vi "disp_dual.vi"(6 "I_B":dbl(slide) scale=0.1..100.0, 7 "I_A":dbl(slide) scale=0.1..100.0, 9 "img_CHB":sgl[][](graph)=array256x256[65536 elements], 10 "img_CHA":sgl[][](graph)=array256x256[65536 elements], 11 "Image Dst":T1) -> (3 "Image":T1(plugin-control))   [LabVIEW 2015]
uses:
  <vilib>/vision/Image Controls.llb/IMAQ Image.ctl
  <vilib>/vision/NI_Vision_Development_Module.lvlib
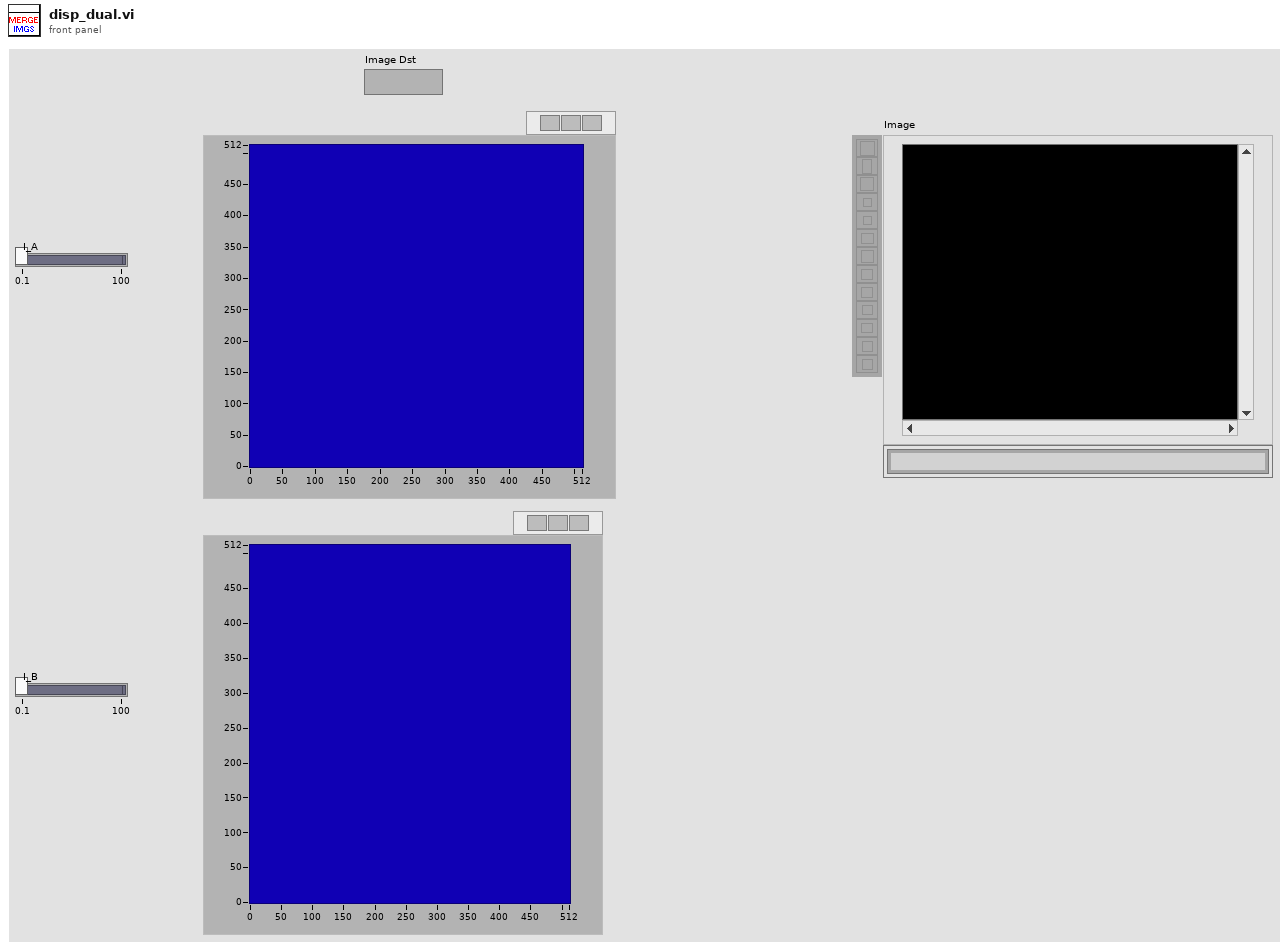
[diagram p1: front panel]
types:
  T1 = typedef "IMAQ Image.ctl" = refnum<image>
  T2 = typedef "Image Type" = u32
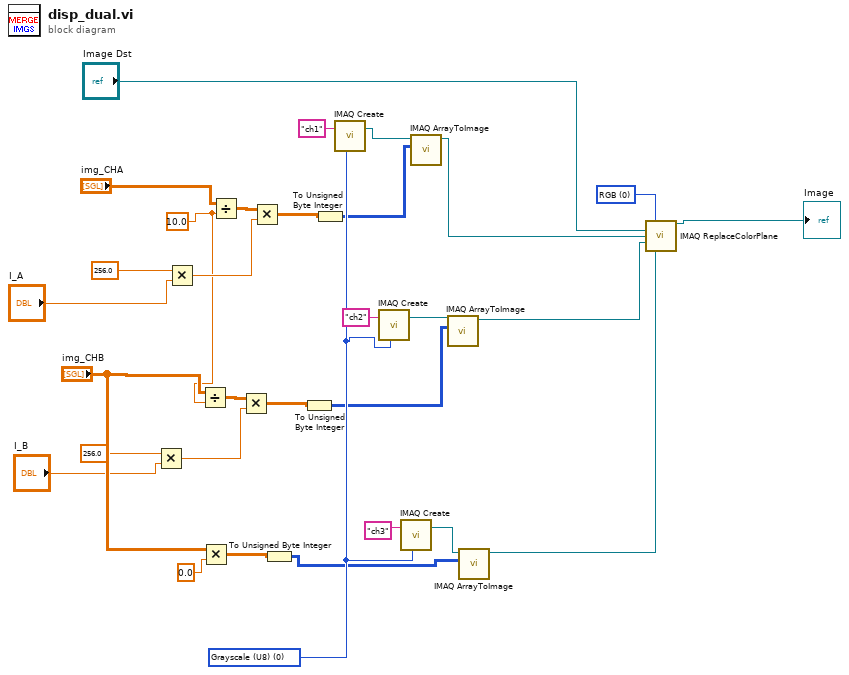
[diagram p0: block diagram]
diagram:
  w1 = 10.0 ("y")
  w21 = T2 0 items=["Grayscale (U8)", "Grayscale (I16)", "Grayscale (SGL)", "Complex (CSG)", "RGB (U32)", "HSL (U32)", "RGB (U64)", "Grayscale (U16)"] ("Image Type")
  w31 = u16 0 items=["RGB", "HSL", "HSV", "HSI"] ("Color Mode")
  n1 = Multiply(x=256.0 ("y"), y="I_B") -> (x*y=w2:dbl)
  n2 = Multiply(x=256.0 ("y"), y="I_A") -> (x*y=w6:dbl)
  n3 = Divide(x="img_CHB", y=w1) -> (x/y=w20:dbl[][])
  n4 = Multiply(x="img_CHB", y=0.0) -> (x*y=w17:dbl[][])
  n5 = Divide(x="img_CHA", y=w1) -> (x/y=w23:dbl[][])
  n6 = Multiply(x=w20, y=w2) -> (x*y=w19:dbl[][])
  n7 = Multiply(x=w23, y=w6) -> (x*y=w22:dbl[][])
  n8 = To Unsigned Byte Integer(number=w17) -> (unsigned 8bit integer=w11:u8[][])
  n9 = To Unsigned Byte Integer(number=w19) -> (unsigned 8bit integer=w9:u8[][])
  n10 = To Unsigned Byte Integer(number=w22) -> (unsigned 8bit integer=w10:u8[][])
  n11 = call "IMAQ Create"("Image Name"="ch1", "Image Type"=w21) -> ("New Image"=w29:T1)  [unwired: 3 in, 1 out]
  n12 = call "IMAQ Create"("Image Name"="ch2", "Image Type"=w21) -> ("New Image"=w28:T1)  [unwired: 3 in, 1 out]
  n13 = call "IMAQ Create"("Image Name"="ch3", "Image Type"=w21) -> ("New Image"=w18:T1)  [unwired: 3 in, 1 out]
  n14 = call "IMAQ ArrayToImage"("Image Pixels (U8)"=w10, "Image"=w29) -> ("Image Out"=w15:T1)  [unwired: 8 in, 1 out]
  n15 = call "IMAQ ArrayToImage"("Image Pixels (U8)"=w9, "Image"=w28) -> ("Image Out"=w14:T1)  [unwired: 8 in, 1 out]
  n16 = call "IMAQ ArrayToImage"("Image Pixels (U8)"=w11, "Image"=w18) -> ("Image Out"=w13:T1)  [unwired: 8 in, 1 out]
  n17 = call "IMAQ ReplaceColorPlane"("Color Mode"=w31, "Image Dst"="Image Dst", "Red or Hue Plane"=w15, "Green or Sat Plane"=w14, "Blue or Luma or Val or Inten Plane"=w13) -> ("Image Dst Out"=→"Image":T1)  [unwired: 9 in, 1 out]
